vi "Write Default to File.vi"(8 "error in (no error)":errorcluster, 9 "Name":string, 10 "Path":path, 11 "Funnel Settings in":refnum<class "Funnel Settings.lvclass">) -> (0 "error out":errorcluster, 3 "Funnel Settings out":refnum<class "Funnel Settings.lvclass">)   [LabVIEW 2019, in "Funnel Settings.lvclass"]
uses:
  Funnel Settings.lvclass
  ObjectSettings/ObjectSettings.lvclass
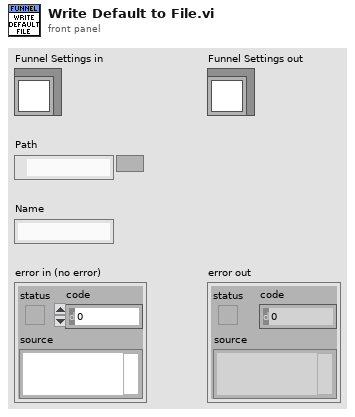
[diagram p1: front panel]
types:
  T1 = typedef "Funnel Settings.lvclass/Default Funnel Cluster.ctl" = cluster{"Smooth Segments":dbl, "Bottom Segments":dbl}
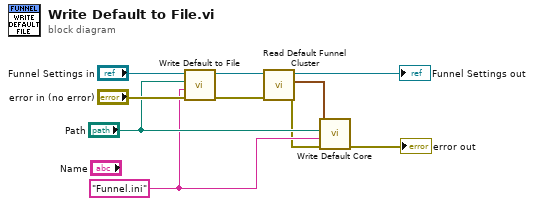
[diagram p0: block diagram]
diagram:
  w4 = "Funnel.ini"
  n1 = call-parent "Write Default to File.vi"("error in (no error)"="error in (no error)", "Name"=w4, "Path"="Path", "ObjectSettings in"="Funnel Settings in") -> ("error out"=w1:errorcluster, "ObjectSettings out"=w8:refnum<class "Funnel Settings.lvclass">)  [unwired: 6 in]
  n2 = call "Read Default Funnel Cluster.vi"("error in (no error)"=w1, "Funnel Settings in"=w8) -> ("error out"=w2:errorcluster, "Default Funnel"=w6:T1, "Funnel Settings out"=→"Funnel Settings out":refnum<class "Funnel Settings.lvclass">)  [unwired: 7 in]
  n3 = call "Write Default Core.vi"("error in (no error)"=w2, "Name"=w4, "Path"="Path", "Cluster In"=w6) -> ("error out"=→"error out":errorcluster)  [unwired: 6 in, 1 out]
